vi "Configure Logic Analyzer Group.vi"(7 "Waveform Size (1: Big)":i32(ring)=1 items=["Small", "Big"], 8 "error in (no error)":errorcluster, 9 "Enable Group State (F: Disable)":bool, 10 "Digital Group (1: Group 1)":i32(ring)=1 items=["Group 1"=1, "Group 2"=2], 11 "VISA resource name":refnum<visa-resource-name>) -> (0 "error out":errorcluster, 3 "VISA resource name out":refnum<visa-resource-name>)   [LabVIEW 2023, in "RIGOL DS1054Z.lvlib"]
doc: "Configures the digital group setttings for logic analyzer.\n\nNote:\nThis VI is only valid for DS1052D and DS1102D."
uses:
  RIGOL DS1054Z.lvlib
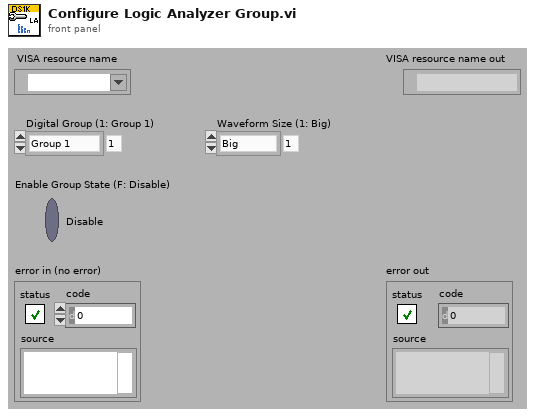
[diagram p1: front panel]
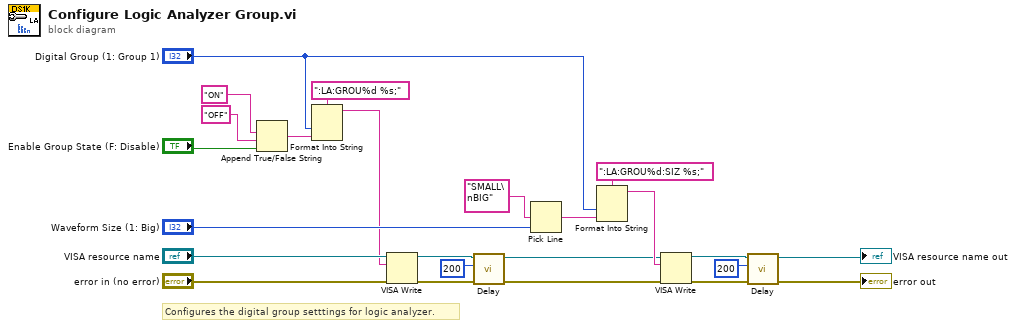
[diagram p0: block diagram]
diagram:
  # "Configures the digital group setttings for logic analyzer."
  n1 = Append True/False String(1:"Enable Group State (F: Disable)", 2:"OFF", 3:"ON") -> (0:w20:string)  [unwired: 1 out]
  n2 = Format Into String(format string=":LA:GROU%d %s;", "Digital Group (1: Group 1)", w20) -> (resulting string=w2:string)  [unwired: 2 in, 1 out]
  n3 = VISA Write(VISA resource name="VISA resource name", write buffer=w2, error in (no error)="error in (no error)") -> (VISA resource name out=w8:refnum<visa-resource-name>, error out=w9:errorcluster)  [unwired: 1 out]
  n4 = call "Delay.vi"("error in (no error)"=w9, "Delay (ms)"=u32 200, "VISA resource name"=w8) -> ("error out"=w3:errorcluster, "VISA resource name out"=w4:refnum<visa-resource-name>)  [unwired: 7 out]
  n5 = Pick Line(multi-line string="SMALL\nBIG", line index="Waveform Size (1: Big)") -> (output string=w16:string)  [unwired: 1 out]
  n6 = Format Into String(format string=":LA:GROU%d:SIZ %s;", "Digital Group (1: Group 1)", w16) -> (resulting string=w15:string)  [unwired: 2 in, 1 out]
  n7 = VISA Write(VISA resource name=w4, write buffer=w15, error in (no error)=w3) -> (VISA resource name out=w13:refnum<visa-resource-name>, error out=w12:errorcluster)  [unwired: 1 out]
  n8 = call "Delay.vi"("error in (no error)"=w12, "Delay (ms)"=u32 200, "VISA resource name"=w13) -> ("error out"=→"error out":errorcluster, "VISA resource name out"=→"VISA resource name out":refnum<visa-resource-name>)  [unwired: 7 out]
